vi "Proporcional.vi"(1 "Kp":dbl, 2 "Error":dbl) -> (0 "Acción Proporcional":dbl)   [LabVIEW 2011]
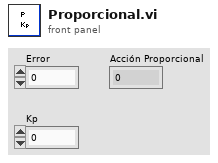
[diagram p1: front panel]
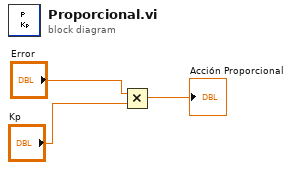
[diagram p0: block diagram]
diagram:
  n1 = Multiply(x="Error", y="Kp") -> (x*y=→"Acción Proporcional":dbl)
